vi "create speedlines UI.vi"() -> (3 "speedlineFile":path)   [LabVIEW 2018]
uses:
  make speedlines UI data.ctl
panel:
  in  "save":bool
  in  "process":bool
  in  "Massflow Channel":u16(ring) items=["time", "gearbox", "Recirculation temp", "volute exit surface", "oil tank", "Inlet average", "Outlet average", "V-cone", "inlet pressure", "outlet pressure", "Motor speed", "V-cone DP", "Motor power", "Accelerometer", "Hotwire", "oil pressure", "butterfly valve position", "ball valve position", "Legacy speed", "new Vcone", "V-Cone: CR001", "pressure ratio", "Ambient pressure", "Ambient temperature"]
  in  "PR Channel":u16(ring) items=["time", "gearbox", "Recirculation temp", "volute exit surface", "oil tank", "Inlet average", "Outlet average", "V-cone", "inlet pressure", "outlet pressure", "Motor speed", "V-cone DP", "Motor power", "Accelerometer", "Hotwire", "oil pressure", "butterfly valve position", "ball valve position", "Legacy speed", "new Vcone", "V-Cone: CR001", "pressure ratio", "Ambient pressure", "Ambient temperature"]
  out "plot":cluster{"mDot":dbl[], "PR":dbl[]}[](graph)
  in  "done":bool
  out "readingFiles":u8(slide) scale=0.0..12.0
  in  "Datafiles":path
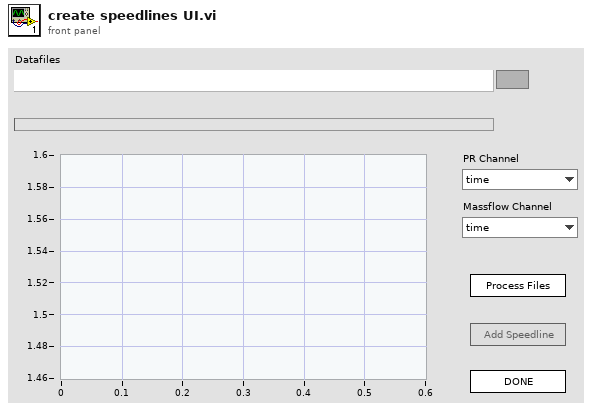
[diagram p1: front panel]
types:
  T1 = enum8{"Enabled", "Disabled", "Disabled and Grayed Out"}
  T2 = typedef "make speedlines UI data.ctl" = cluster{"folder":path, "PR Channel":u16, "Massflow Channel":u16, "speedlineCount":u16, "massFlowData":dbl[], "PRdata":dbl[], "progress":refnum<vi>, "PR":refnum<vi>, "massflow":refnum<vi>, "speedlineFileRef":refnum<file>, "speedlineFile":path, "speedlines":cluster{"mDot":dbl[], "PR":dbl[]}[]}
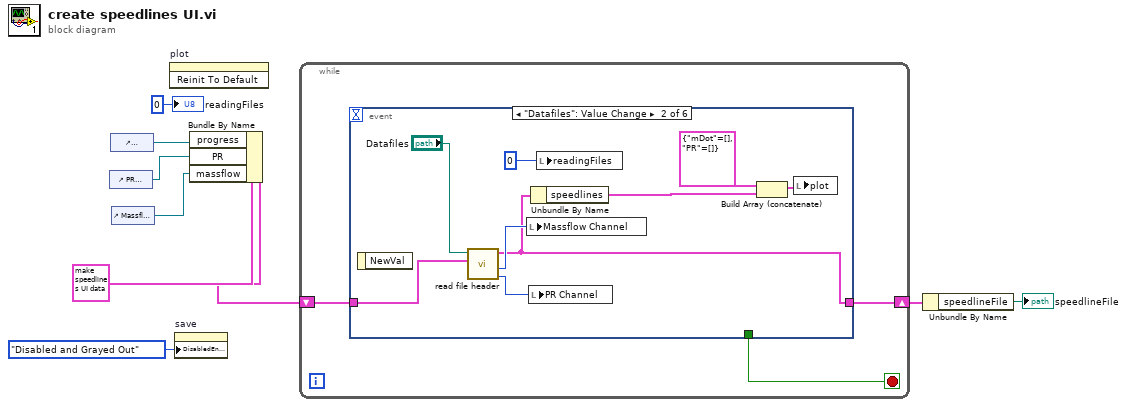
[diagram p0: block diagram]
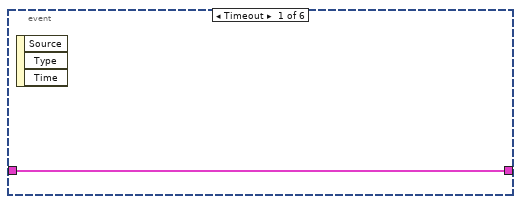
[diagram p2: hidden frame]
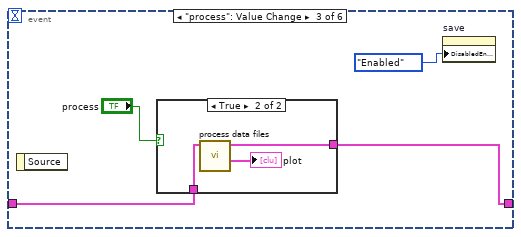
[diagram p3: hidden frame]
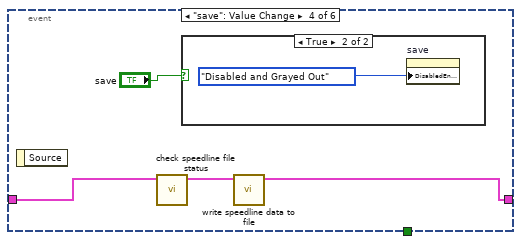
[diagram p5: hidden frame]
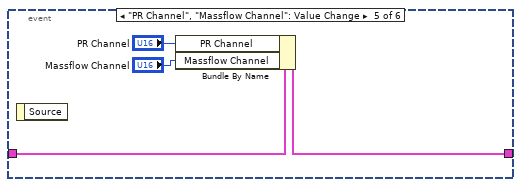
[diagram p7: hidden frame]
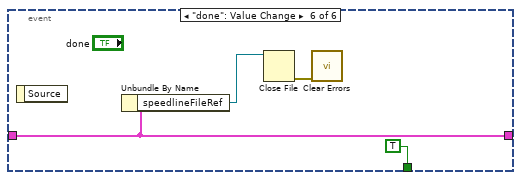
[diagram p8: hidden frame]
diagram:
  n1 = control-ref of="PR Channel"() -> (w6:refnum<vi>)
  n2 = control-ref of="readingFiles"() -> (w7:refnum<vi>)
  n3 = control-ref of="Massflow Channel"() -> (w5:refnum<vi>)
  n4 = invoke on="plot" class="XYGraph (strict)" method="Reinit To Default"() -> ()  [unwired: 3 in, 3 out]
  n5 = property on="save" class="Bool"("DisabledEnum"=T1."Disabled and Grayed Out" ("Disabled")) -> ()  [unwired: 2 in, 2 out]
  n6 = Bundle By Name(cluster=T2 {"folder"=path "", "PR Channel"=0, "Massflow Channel"=0, "speedlineCount"=0, "massFlowData"=[], "PRdata"=[], "progress"=refnum, "PR"=refnum, "massflow"=refnum, "speedlineFileRef"=refnum, "speedlineFile"=path "", "speedlines"=[]}, "progress"=w7, "PR"=w6, "massflow"=w5) -> (w8:T2)
  n7 = while {
    shift-right: [w11] -> w2
    shift-left: w8 -> [w12]
    stop <- w10 stop-if-true
    n8 = event shown="[1] \"Datafiles\": Value Change" {
      selector: _ -> [_ _ _ _ _ _]
      dyn-events: _ -> [_ _ _ _ _ _]
      timeout: _ -> [_ _ _ _ _ _]
      tunnel: w12 -> [w13 w22 w26 w34 w39 w42]
      tunnel: [w13 w17 w25 w32 w38 w42] -> w11
      tunnel: [_ _ _ _ _ TRUE] -> w10
      event Timeout {
        n9 = event-data() -> ()  [unwired: 1 in, 3 out]
      }
      event "Datafiles": Value Change {
        n10 = event-data() -> ()  [unwired: 1 in, 1 out]
        n11 = call "read file header.vi"("makeSpeedlinesData in"=w22, "Datafiles"="Datafiles") -> ("PR"=w19:i32, "massflow"=w20:i32, "makeSpeedlinesData out"=w17:T2)  [unwired: 7 in]
        n12 = local write "Massflow Channel"(w20) -> ()
        n13 = local write "PR Channel"(w19) -> ()
        n14 = Unbundle By Name(w17) -> ("speedlines"=w16:cluster{"mDot":dbl[], "PR":dbl[]}[])
        n15 = local write "readingFiles"(u8 0 ("readingFiles")) -> ()
        n16 = Build Array (concatenate)(cluster{"mDot":dbl[], "PR":dbl[]} {"mDot"=[], "PR"=[]} ("element"), w16) -> (w15:cluster{"mDot":dbl[], "PR":dbl[]}[])
        n17 = local write "plot"(w15) -> ()
      }
      event "process": Value Change {
        n18 = event-data() -> ()  [unwired: 1 in, 1 out]
        n19 = case shown="True" "process" {
          tunnel: w26 -> [w27 w30]
          tunnel: [w27 w29] -> w25
          frame False {
          }
          frame True {
            n20 = call "process data files.vi"("makeSpeedlinesData in"=w30) -> ("appended array"=→"plot":cluster{"mDot":dbl[], "PR":dbl[]}[], "makeSpeedlinesData out"=w29:T2)  [unwired: 9 in]
          }
        }
        n21 = property on="save" class="Bool"("DisabledEnum"=T1."Enabled" ("Disabled")) -> ()  [unwired: 2 in, 2 out]
      }
      event "save": Value Change {
        n22 = event-data() -> ()  [unwired: 1 in, 1 out]
        n23 = call "check speedline file status.vi"("makeSpeedlinesData in"=w34) -> ("makeSpeedlinesData out"=w33:T2)  [unwired: 10 in]
        n24 = case shown="True" "save" {
          frame False {
          }
          frame True {
            n25 = property on="save" class="Bool"("DisabledEnum"=T1."Disabled and Grayed Out" ("Disabled")) -> ()  [unwired: 2 in, 2 out]
          }
        }
        n26 = call "write speedline data to file.vi"("makeSpeedlinesData in"=w33) -> ("makeSpeedlinesData out"=w32:T2)  [unwired: 10 in]
      }
      event "PR Channel", "Massflow Channel": Value Change {
        n27 = event-data() -> ()  [unwired: 1 in, 1 out]
        n28 = Bundle By Name(cluster=w39, "PR Channel"="PR Channel", "Massflow Channel"="Massflow Channel") -> (w38:T2)
      }
      event "done": Value Change {
        n29 = event-data() -> ()  [unwired: 1 in, 1 out]
        n30 = Unbundle By Name(w42) -> ("speedlineFileRef"=w41:refnum<file>)
        n31 = Close File(refnum=w41) -> (error out=w40:errorcluster)  [unwired: 1 in, 1 out]
        n32 = call <vilib>:"Clear Errors.vi"("error in (no error)"=w40) -> ()  [unwired: 5 in, 2 out]
      }
    }
  }
  n33 = Unbundle By Name(w2) -> ("speedlineFile"=→"speedlineFile":path)
  "readingFiles" <- u8 0 ("readingFiles")
